vi "SE5082_Configure_waveform.vi"(8 "error in":errorcluster, 9 "Channel":u16(ring)=1 items=["Channel 1", "Channel 2"], 10 "Sampling rate":i64=5000000000, 11 "VISA resource name in":refnum<visa-resource-name>="USB0::0x168C::0x5082::0000217419::INSTR") -> (0 "error out":errorcluster, 3 "VISA resource name out":refnum<visa-resource-name>="USB0::0x168C::0x5082::0000217419::INSTR")   [LabVIEW 2017]
panel:
  in  "Readout status?":bool
  in  "Read-out commands":string[](array[string])=[":INIT:CONT?", ":TRIG:SOUR:ADV?", ":FREQ:RAST?"]
  out "Input waveform commands":string[](array[string])=[":INST:SEL 2", ":INIT:CONT OFF", ":TRIG:COUN 1", ":TRIG:DEL 0", ":TRIG:LEV 1.5", ":TRIG:MODE NORM", ":TRIG:SLOP POS", ":TRIG:SOUR:ADV EXT", ":TRIG:BURS ON", ":TRIG:STATE ON", ":FREQ:RAST 5000000000"]
  out "Status output":string[](array[string])=["OFF\n", "EXT\n", "5.000000000e+09\n"]
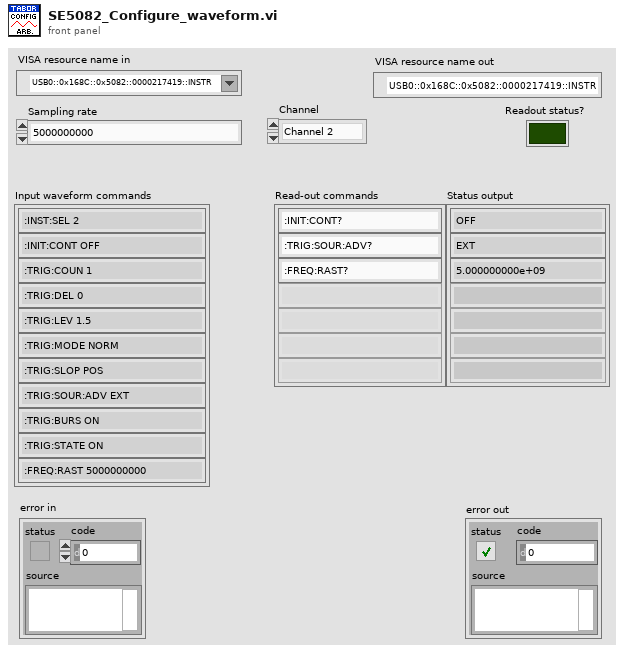
[diagram p1: front panel]
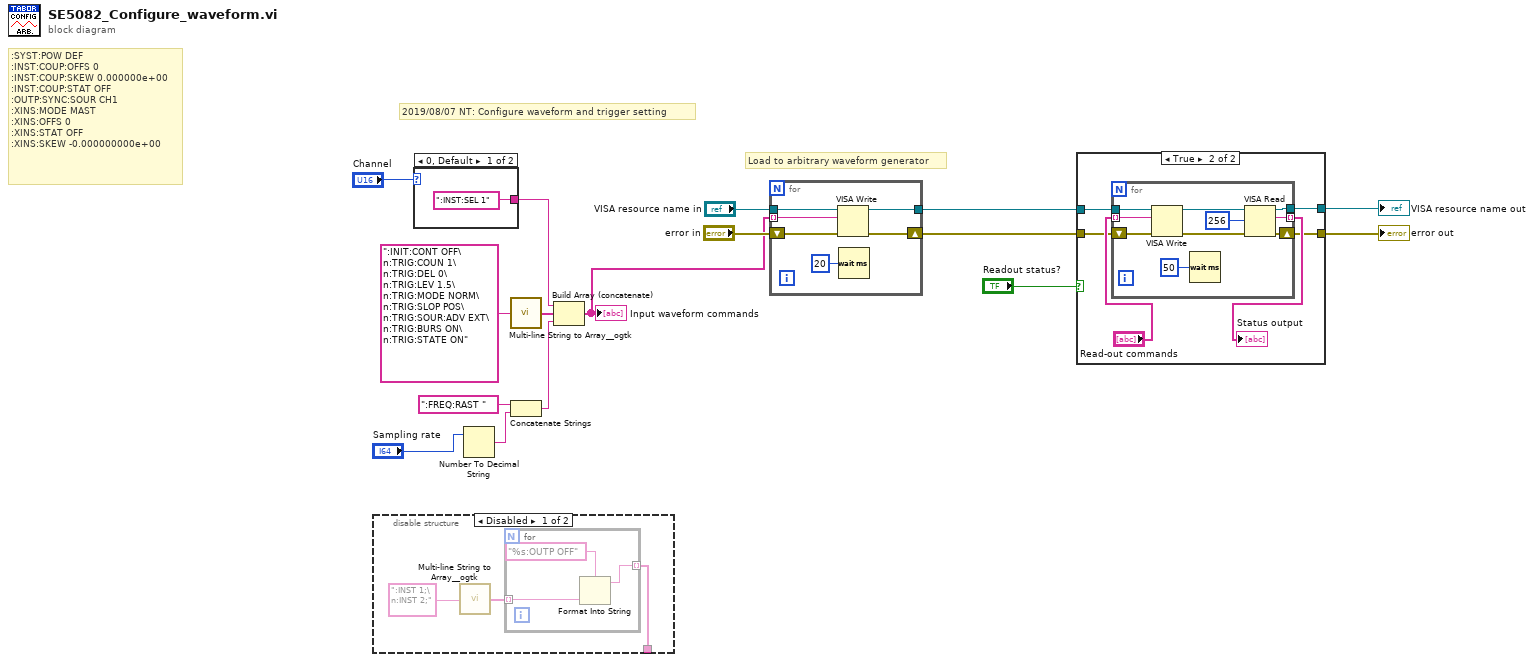
[diagram p0: block diagram]
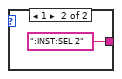
[diagram p3: hidden frame]
diagram:
  # ":SYST:POW DEF\n:INST:COUP:OFFS 0\n:INST:COUP:SKEW 0.000000e+00\n:INST:COUP:STAT OFF\n:OUTP:SYNC:SOUR CH1\n:XINS:MODE MAST\n:XINS:OFFS 0\n:XINS:STAT OFF\n:XINS:SKEW -0.000000000e+00"
  # "2019/08/07 NT: Configure waveform and trigger setting"
  # "Load to arbitrary waveform generator"
  n1 = disable-structure shown="Disabled" {
    disable-tunnel: [w17 _] -> _
    frame Disabled {
      n2 = call <userlib>:"Multi-line String to Array__ogtk.vi"("string"=":INST 1;\n:INST 2;" ("initial string")) -> ("lines"=w18:string[])
      n3 = for {
        tunnel: w18 -> [w20] mode=indexing
        tunnel: [w21] -> w17 mode=indexing
        n4 = Format Into String(format string="%s:OUTP OFF", w20) -> (resulting string=w21:string)  [unwired: 2 in, 1 out]
      }
    }
    frame Enabled {
    }
  }
  n5 = case shown="0, Default" "Channel" {
    tunnel: [":INST:SEL 1" ("initial string") ":INST:SEL 2" ("initial string")] -> w6
    frame 0, Default {
    }
    frame 1 {
    }
  }
  n6 = Number To Decimal String(number="Sampling rate") -> (decimal integer string=w8:string)  [unwired: 1 in]
  n7 = call <userlib>:"Multi-line String to Array__ogtk.vi"("string"=":INIT:CONT OFF\n:TRIG:COUN 1\n:TRIG:DEL 0\n:TRIG:LEV 1.5\n:TRIG:MODE NORM\n:TRIG:SLOP POS\n:TRIG:SOUR:ADV EXT\n:TRIG:BURS ON\n:TRIG:STATE ON" ("write buffer")) -> ("lines"=w2:string[])
  n8 = Concatenate Strings(":FREQ:RAST ", w8) -> (w1:string)
  n9 = Build Array (concatenate)(w6, w2, w1) -> (w3:string[])
  "Input waveform commands" <- w3
  n10 = for {
    tunnel: "VISA resource name in" -> [w30]
    tunnel: w3 -> [w25] mode=indexing
    shift-right: [w28] -> w14
    shift-left: "error in" -> [w29]
    tunnel: [w27] -> w15
    n11 = VISA Write(VISA resource name=w30, write buffer=w25, error in (no error)=w29) -> (VISA resource name out=w27:refnum<visa-resource-name>, error out=w28:errorcluster)  [unwired: 1 out]
    n12 = Wait (ms)(milliseconds to wait=u32 20) -> ()  [unwired: 1 out]
  }
  n13 = case shown="True" "Readout status?" {
    tunnel: w15 -> [w32 w36]
    tunnel: w14 -> [w31 w35]
    tunnel: [w31 w34] -> w13
    tunnel: [w32 w33] -> w12
    frame False {
    }
    frame True {
      n14 = for {
        tunnel: [w45] -> w38 mode=indexing
        shift-right: [w44] -> w34
        shift-left: w35 -> [w41]
        tunnel: w36 -> [w43]
        tunnel: "Read-out commands" -> [w42] mode=indexing
        tunnel: [w39] -> w33
        n15 = VISA Write(VISA resource name=w43, write buffer=w42, error in (no error)=w41) -> (VISA resource name out=w47:refnum<visa-resource-name>, error out=w46:errorcluster)  [unwired: 1 out]
        n16 = Wait (ms)(milliseconds to wait=u32 50) -> ()  [unwired: 1 out]
        n17 = VISA Read(VISA resource name=w47, byte count=u32 256, error in (no error)=w46) -> (VISA resource name out=w39:refnum<visa-resource-name>, read buffer=w45:string, error out=w44:errorcluster)  [unwired: 1 out]
      }
      "Status output" <- w38
    }
  }
  "error out" <- w13
  "VISA resource name out" <- w12
